vi "Properties_Dotted_Prepend Parent ID and Label.vi"(9 "Parent Name":string, 10 "Parent ID":string, 11 "Property Arr In":T1(array[cluster])) -> (3 "Property Arr Out":T1(array[cluster]))   [LabVIEW 2023]
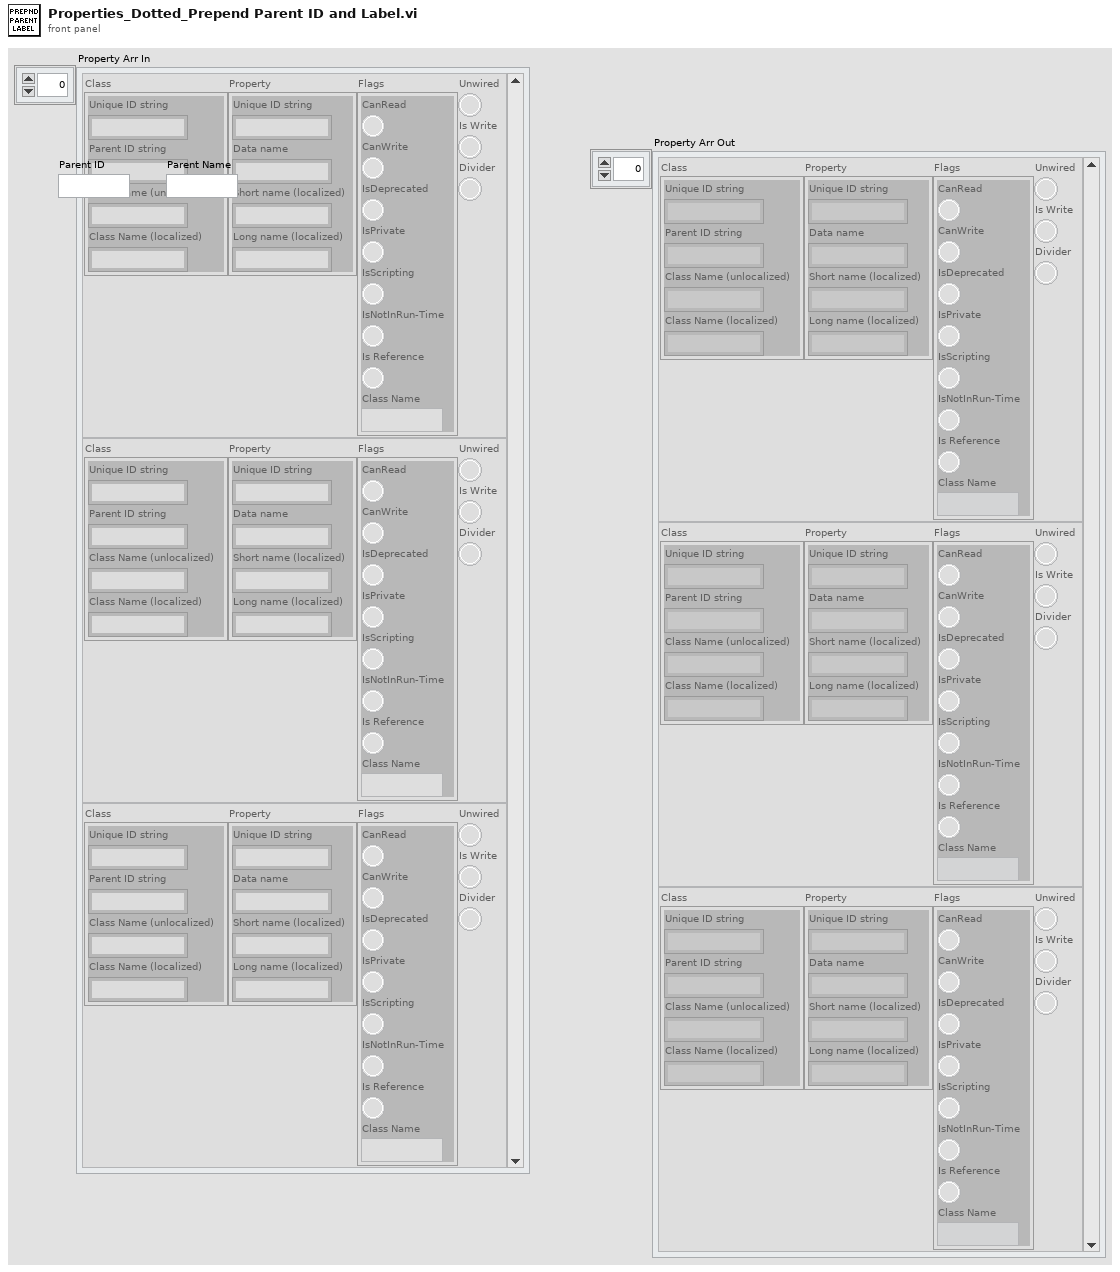
[diagram p1: front panel]
types:
  T1 = cluster{"Class":cluster{"Unique ID string":string, "Parent ID string":string, "Class Name (unlocalized)":string, "Class Name (localized)":string}, "Property":cluster{"Unique ID string":string, "Data name":string, "Short name (localized)":string, "Long name (localized)":string}, "Flags":cluster{"CanRead":bool, "CanWrite":bool, "IsDeprecated":bool, "IsPrivate":bool, "IsScripting":bool, "IsNotInRun-Time":bool, "Is Reference":bool, "Class Name":string}, "Divider":bool, "Is Write":bool, "Unwired":bool}[]
  T2 = cluster{"Class":cluster{"Unique ID string":string, "Parent ID string":string, "Class Name (unlocalized)":string, "Class Name (localized)":string}, "Property":cluster{"Unique ID string":string, "Data name":string, "Short name (localized)":string, "Long name (localized)":string}, "Flags":cluster{"CanRead":bool, "CanWrite":bool, "IsDeprecated":bool, "IsPrivate":bool, "IsScripting":bool, "IsNotInRun-Time":bool, "Is Reference":bool, "Class Name":string}, "Divider":bool, "Is Write":bool, "Unwired":bool}
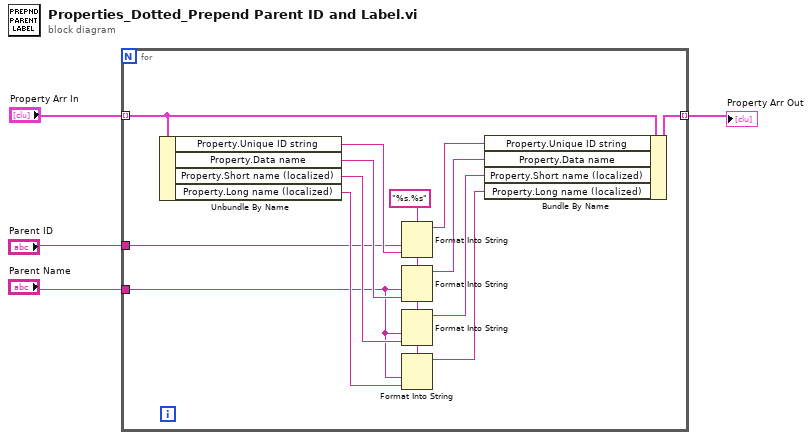
[diagram p0: block diagram]
diagram:
  n1 = for {
    tunnel: [w16] -> w4 mode=indexing
    tunnel: "Property Arr In" -> [w17] mode=indexing
    tunnel: "Parent ID" -> [w11]
    tunnel: "Parent Name" -> [w10]
    w9 = "%s.%s" ("format string")
    n2 = Unbundle By Name(w17) -> ("Property.Unique ID string"=w15:string, "Property.Data name"=w14:string, "Property.Short name (localized)"=w13:string, "Property.Long name (localized)"=w12:string)
    n3 = Format Into String(format string=w9, w11, w15) -> (resulting string=w8:string)  [unwired: 2 in, 1 out]
    n4 = Format Into String(format string=w9, w10, w14) -> (resulting string=w7:string)  [unwired: 2 in, 1 out]
    n5 = Format Into String(format string=w9, w10, w13) -> (resulting string=w6:string)  [unwired: 2 in, 1 out]
    n6 = Format Into String(format string=w9, w10, w12) -> (resulting string=w5:string)  [unwired: 2 in, 1 out]
    n7 = Bundle By Name(cluster=w17, "Property.Unique ID string"=w8, "Property.Data name"=w7, "Property.Short name (localized)"=w6, "Property.Long name (localized)"=w5) -> (w16:T2)
  }
  "Property Arr Out" <- w4
